vi "TDMS Get Display Settings.vi"(8 "error in (no error)":errorcluster, 10 "Run String":string="Run 1", 11 "TDM File Path":path) -> (0 "error out":errorcluster, 3 "Parameters":T1)   [LabVIEW 2011]
uses:
  ITK EXT/utils/keyedarr.llb/Keyed Array.ctl
  ITK EXT/utils/strutil.llb/Case Matching.ctl
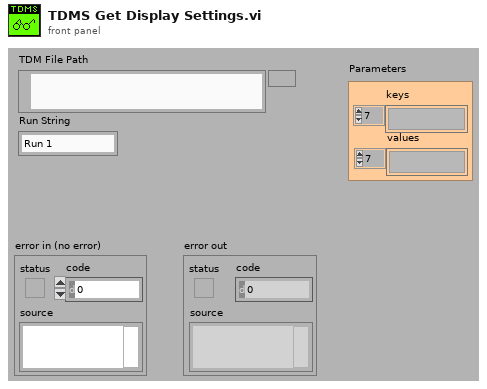
[diagram p1: front panel]
types:
  T1 = typedef "Keyed Array.ctl" = cluster{"keys":string[], "values":string[]}
  T2 = typedef "Case Matching.ctl" = enum16{"a != A", "a == A", "system"}
  T3 = enum16{"open", "open or create", "create or replace", "create", "open (read-only)"}
  T4 = typedef "Field Record.ctl" = cluster{"ixField":i32, "iSequenceOrder":i32, "sxFieldId":string, "sxSequenceId":string, "sDisplayName":string, "sValue":string, "sUnits":string, "nDataType":T5, "nNextItem":T6, "fSystem":bool, "fSystemValue":bool, "fRequired":bool, "fSetAtTest":bool, "fTestField":bool, "fDeleted":bool, "fIndexed":bool, "fFreeList":bool}
  T5 = typedef "Field DataTypes.ctl" = enum32{"text", "numeric", "list", "timestamp", "boolean"}
  T6 = typedef "Field NextItem.ctl" = enum32{"Reset", "Retain", "Auto-Increment"}
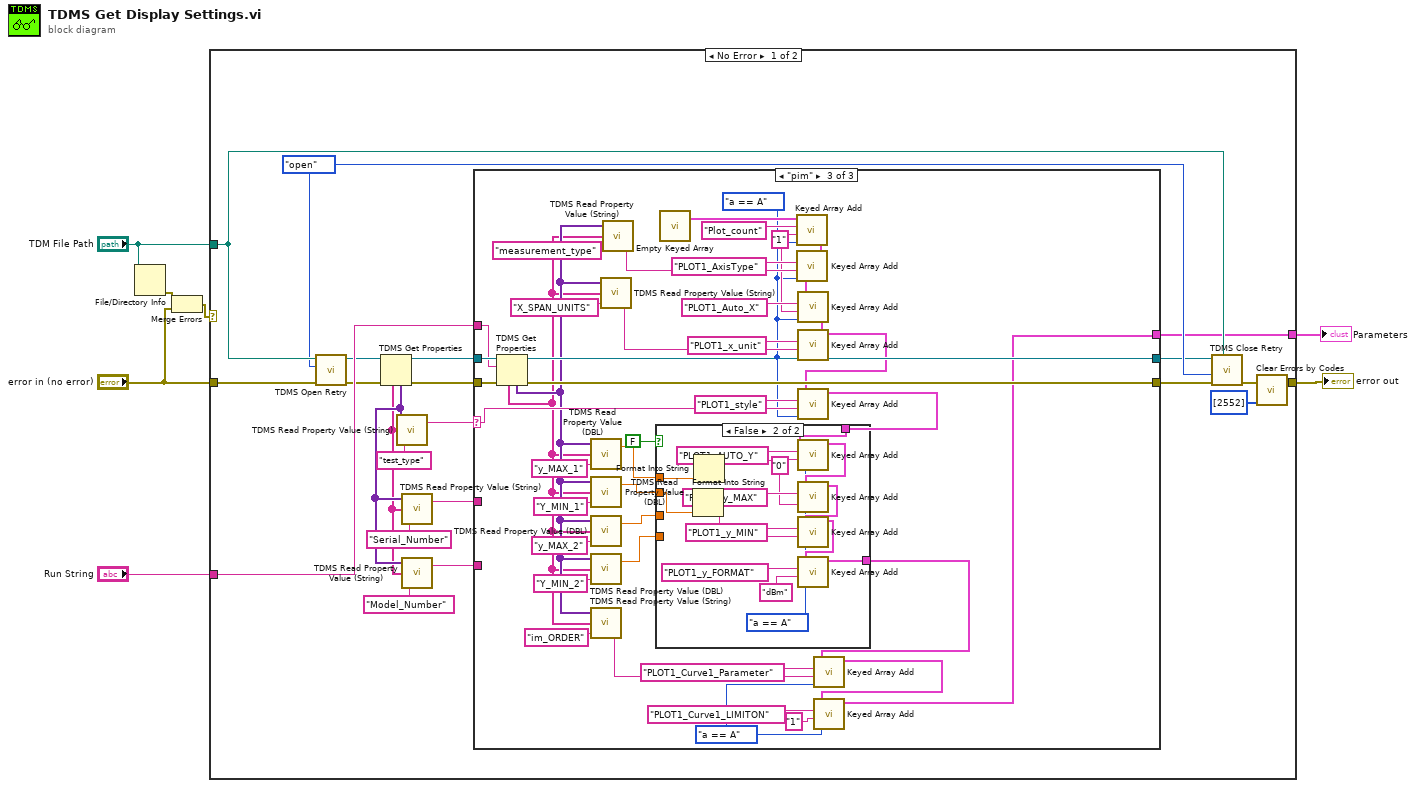
[diagram p0: block diagram]
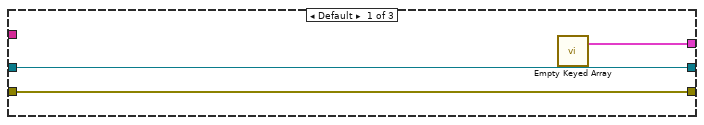
[diagram p2: hidden frame]
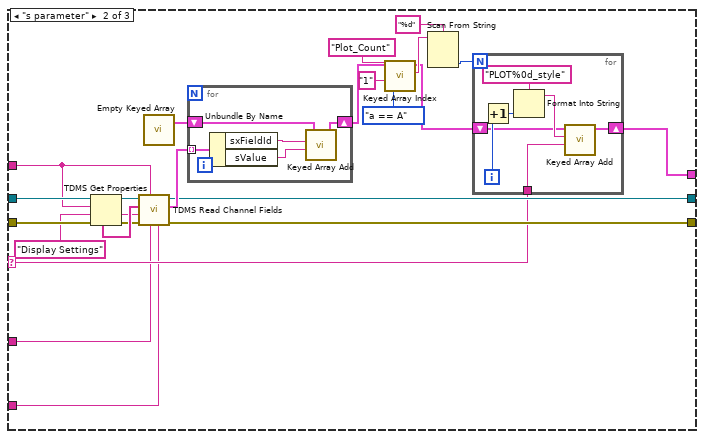
[diagram p3: hidden frame]
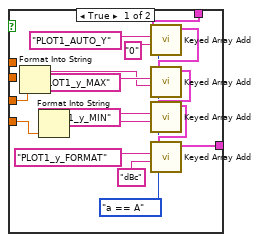
[diagram p4: hidden frame]
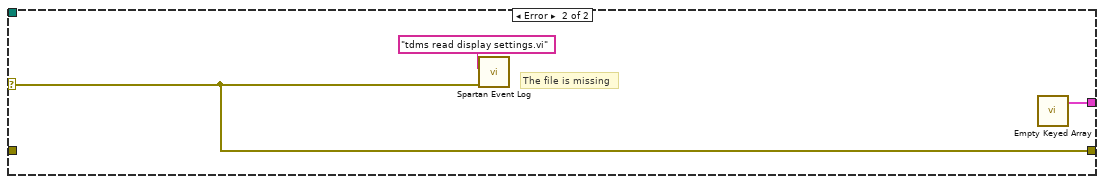
[diagram p5: hidden frame]
diagram:
  n1 = File/Directory Info(path="TDM File Path") -> (error out=w6:errorcluster)  [unwired: 1 in, 6 out]
  n2 = Merge Errors(w6, "error in (no error)") -> (w4:errorcluster)
  n3 = case shown="No Error" w4 {
    selector: w4 -> [_ w142]
    tunnel: [w25 w142] -> w2
    tunnel: "error in (no error)" -> [w9 _]
    tunnel: "TDM File Path" -> [w29 _]
    tunnel: "Run String" -> [w24 _]
    tunnel: [w17 w143] -> w1
    frame No Error {
      w28 = T3."open" ("operation (0:open)")
      n4 = call "TDMS Open Retry.vi"("error in (no error)"=w9, "Operation (0:open)"=w28, "Path"=w29) -> ("error out"=w21:errorcluster, "TDMS File Ref"=w22:refnum<k34>)  [unwired: 1 in, 6 out]
      n5 = TDMS Get Properties(8:w21, 11:w22) -> (0:w19:errorcluster, 3:w20:refnum<k34>, 4:w14:variant[], 6:w8:string[])  [unwired: 6 out]
      n6 = call "TDMS Read Property Value (String).vi"("Property Name"="test_type", "Property Names"=w8, "Property Values"=w14) -> ("Property Value"=w18:string)  [unwired: 1 out]
      n7 = call "TDMS Read Property Value (String).vi"("Property Name"="Serial_Number" ("sxFieldId"), "Property Names"=w8, "Property Values"=w14) -> ("Property Value"=w11:string)  [unwired: 1 out]
      n8 = call "TDMS Read Property Value (String).vi"("Property Name"="Model_Number" ("sxFieldId"), "Property Names"=w8, "Property Values"=w14) -> ("Property Value"=w10:string)  [unwired: 1 out]
      n9 = case shown="\"pim\"" w18 {
        selector: w18 -> [_ w44 w85]
        tunnel: w24 -> [_ w45 w107]
        tunnel: w20 -> [w31 w54 w110]
        tunnel: w19 -> [w30 w53 w109]
        tunnel: [w32 w35 w73] -> w17
        tunnel: [w31 w47 w105] -> w16
        tunnel: [w30 w46 w104] -> w15
        tunnel: w11 -> [_ w34 _]
        tunnel: w10 -> [_ w33 _]
        frame Default {
          n10 = call "Empty Keyed Array.vi"() -> ("empty keyed array"=w32:T1)  [unwired: 3 out]
        }
        frame "s parameter" {
          w51 = "Display Settings" ("Property Name")
          n11 = TDMS Get Properties(8:w53, 9:w51, 10:w45, 11:w54) -> (0:w52:errorcluster, 3:w50:refnum<k34>, 6:w55:string[])  [unwired: 5 out]
          n12 = call "TDMS Read Channel Fields.vi"("MN"=w33, "SN"=w34, "Group Name"=w45, "error in (no error)"=w52, "Channel"=w51, "Custom Field Records to Search"=w55, "tdms file ref"=w50) -> ("error out"=w46:errorcluster, "Custom Fields"=w49:T4[], "tdms file ref"=w47:refnum<k34>)  [unwired: 2 in]
          n13 = call "Empty Keyed Array.vi"() -> ("empty keyed array"=w48:T1)  [unwired: 3 out]
          n14 = for {
            tunnel: w49 -> [w67] mode=indexing
            shift-right: [w63] -> w40
            shift-left: w48 -> [w66]
            n15 = Unbundle By Name(w67) -> ("sxFieldId"=w65:string, "sValue"=w64:string)
            n16 = call "Keyed Array Add.vi"("value"=w64, "key"=w65, "array in"=w66) -> ("array out"=w63:T1)  [unwired: 1 in, 3 out]
          }
          n17 = call "Keyed Array Index.vi"("case matching (sensitive)"=Case_Matching."a == A", "default value"="1", "key"="Plot_Count" ("format string"), "array in"=w40) -> ("value"=w38:string, "duplicate array"=w36:T1)  [unwired: 2 out]
          n18 = Scan From String(format string="%d", input string=w38) -> (output 1=w39:i32)  [unwired: 2 in, 4 out]
          n19 = for {
            N: w39 -> [_]
            tunnel: w44 -> [w62]
            shift-right: [w56] -> w35
            shift-left: w36 -> [w57]
            i -> [w59]
            n20 = Increment(x=w59) -> (x+1=w58:i32)
            n21 = Format Into String(format string="PLOT%0d_style" ("Property Name"), w58) -> (resulting string=w60:string)  [unwired: 2 in, 1 out]
            n22 = call "Keyed Array Add.vi"("value"=w62, "key"=w60, "array in"=w57) -> ("array out"=w56:T1)  [unwired: 1 in, 3 out]
          }
        }
        frame "pim" {
          w74 = Case_Matching."a == A" ("case matching (sensitive)")
          w75 = Case_Matching."a == A" ("case matching (sensitive)")
          w97 = "1" ("Property Name")
          n23 = TDMS Get Properties(8:w109, 10:w107, 11:w110) -> (0:w104:errorcluster, 3:w105:refnum<k34>, 4:w81:variant[], 6:w80:string[])  [unwired: 5 out]
          n24 = call "TDMS Read Property Value (DBL).vi"("Property Name"="y_MAX_1", "Property Names"=w80, "Property Values"=w81) -> ("Property Value"=w71:dbl)  [unwired: 1 out]
          n25 = call "TDMS Read Property Value (DBL).vi"("Property Name"="Y_MIN_1", "Property Names"=w80, "Property Values"=w81) -> ("Property Value"=w70:dbl)  [unwired: 1 out]
          n26 = call "TDMS Read Property Value (DBL).vi"("Property Name"="y_MAX_2", "Property Names"=w80, "Property Values"=w81) -> ("Property Value"=w69:dbl)  [unwired: 1 out]
          n27 = call "TDMS Read Property Value (DBL).vi"("Property Name"="Y_MIN_2", "Property Names"=w80, "Property Values"=w81) -> ("Property Value"=w68:dbl)  [unwired: 1 out]
          n28 = call "TDMS Read Property Value (String).vi"("Property Name"="im_ORDER", "Property Names"=w80, "Property Values"=w81) -> ("Property Value"=w79:string)  [unwired: 1 out]
          n29 = call "TDMS Read Property Value (String).vi"("Property Name"="X_SPAN_UNITS", "Property Names"=w80, "Property Values"=w81) -> ("Property Value"=w93:string)  [unwired: 1 out]
          n30 = call "TDMS Read Property Value (String).vi"("Property Name"="measurement_type", "Property Names"=w80, "Property Values"=w81) -> ("Property Value"=w102:string)  [unwired: 1 out]
          n31 = call "Empty Keyed Array.vi"() -> ("empty keyed array"=w108:T1)  [unwired: 3 out]
          n32 = call "Keyed Array Add.vi"("case matching (sensitive)"=w74, "value"=w97, "key"="Plot_count" ("Property Name"), "array in"=w108) -> ("array out"=w100:T1)  [unwired: 3 out]
          n33 = call "Keyed Array Add.vi"("case matching (sensitive)"=w74, "value"=w102, "key"="PLOT1_AxisType" ("Property Name"), "array in"=w100) -> ("array out"=w99:T1)  [unwired: 3 out]
          n34 = call "Keyed Array Add.vi"("case matching (sensitive)"=w74, "value"=w97, "key"="PLOT1_Auto_X" ("Property Name"), "array in"=w99) -> ("array out"=w96:T1)  [unwired: 3 out]
          n35 = call "Keyed Array Add.vi"("case matching (sensitive)"=w74, "value"=w93, "key"="PLOT1_x_unit" ("Property Name"), "array in"=w96) -> ("array out"=w86:T1)  [unwired: 3 out]
          n36 = call "Keyed Array Add.vi"("case matching (sensitive)"=w74, "value"=w85, "key"="PLOT1_style" ("Property Name"), "array in"=w86) -> ("array out"=w87:T1)  [unwired: 3 out]
          n37 = case shown="False" FALSE {
            tunnel: w69 -> [w111 _]
            tunnel: w68 -> [w114 _]
            tunnel: w87 -> [w116 w131]
            tunnel: w71 -> [_ w129]
            tunnel: w70 -> [_ w127]
            tunnel: [w115 w130] -> w84
            frame True {
              w117 = Case_Matching."a == A" ("case matching (sensitive)")
              w113 = "PLOT1_y_MIN" ("Property Name")
              n38 = Format Into String(w111) -> (resulting string=w112:string)  [unwired: 3 in, 1 out]
              n39 = Format Into String(w114) -> ()  [unwired: 3 in, 2 out]
              n40 = call "Keyed Array Add.vi"("case matching (sensitive)"=w117, "value"="0" ("Property Name"), "key"="PLOT1_AUTO_Y" ("Property Name"), "array in"=w116) -> ("array out"=w120:T1)  [unwired: 3 out]
              n41 = call "Keyed Array Add.vi"("case matching (sensitive)"=w117, "value"=w112, "key"="PLOT1_y_MAX" ("Property Name"), "array in"=w120) -> ("array out"=w119:T1)  [unwired: 3 out]
              n42 = call "Keyed Array Add.vi"("case matching (sensitive)"=w117, "value"=w113, "key"=w113, "array in"=w119) -> ("array out"=w118:T1)  [unwired: 3 out]
              n43 = call "Keyed Array Add.vi"("case matching (sensitive)"=w117, "value"="dBc" ("Property Name"), "key"="PLOT1_y_FORMAT" ("Property Name"), "array in"=w118) -> ("array out"=w115:T1)  [unwired: 3 out]
            }
            frame False {
              w132 = Case_Matching."a == A" ("case matching (sensitive)")
              n44 = Format Into String(w127) -> (resulting string=w126:string)  [unwired: 3 in, 1 out]
              n45 = Format Into String(w129) -> (resulting string=w128:string)  [unwired: 3 in, 1 out]
              n46 = call "Keyed Array Add.vi"("case matching (sensitive)"=w132, "value"="0" ("Property Name"), "key"="PLOT1_AUTO_Y" ("Property Name"), "array in"=w131) -> ("array out"=w135:T1)  [unwired: 3 out]
              n47 = call "Keyed Array Add.vi"("case matching (sensitive)"=w132, "value"=w128, "key"="PLOT1_y_MAX" ("Property Name"), "array in"=w135) -> ("array out"=w134:T1)  [unwired: 3 out]
              n48 = call "Keyed Array Add.vi"("case matching (sensitive)"=w132, "value"=w126, "key"="PLOT1_y_MIN" ("Property Name"), "array in"=w134) -> ("array out"=w133:T1)  [unwired: 3 out]
              n49 = call "Keyed Array Add.vi"("case matching (sensitive)"=w132, "value"="dBm" ("Property Name"), "key"="PLOT1_y_FORMAT" ("Property Name"), "array in"=w133) -> ("array out"=w130:T1)  [unwired: 3 out]
            }
          }
          n50 = call "Keyed Array Add.vi"("case matching (sensitive)"=w75, "value"=w79, "key"="PLOT1_Curve1_Parameter" ("Property Name"), "array in"=w84) -> ("array out"=w78:T1)  [unwired: 3 out]
          n51 = call "Keyed Array Add.vi"("case matching (sensitive)"=w75, "value"="1" ("Property Name"), "key"="PLOT1_Curve1_LIMITON" ("Property Name"), "array in"=w78) -> ("array out"=w73:T1)  [unwired: 3 out]
        }
      }
      n52 = call "TDMS Close Retry.vi"("TDMS Path"=w29, "error in (no error)"=w15, "Operation (0:open)"=w28, "TDMS File Ref"=w16) -> ("error out"=w26:errorcluster)  [unwired: 1 in, 6 out]
      n53 = call "Clear Errors by Codes.vi"("Error Codes\nto Clear (Empty)"=i32[] [2552] ("Error Codes\nto Clear (Empty)"), "error in (no error)"=w26) -> ("error out"=w25:errorcluster)  [unwired: 5 out]
    }
    frame Error {
      # "The file is missing"
      n54 = call "Spartan Event Log.vi"("error in (no error)"=w142, "module (\"\")"="tdms read display settings.vi") -> ()  [unwired: 6 in, 1 out]
      n55 = call "Empty Keyed Array.vi"() -> ("empty keyed array"=w143:T1)  [unwired: 3 out]
    }
  }
  "error out" <- w2
  "Parameters" <- w1
